vi "dlgTVEFeRFePlot.vi"(8 "error in (no error)":errorcluster, 11 "ResultArray":T1 {"Time Stamp" format="%^<%.3X\n%x>T"}) -> (0 "error out":errorcluster)   [LabVIEW 2014]
uses:
  typedefs/PlotSource.ctl
  typedefs/ResultArray.ctl
  typedefs/Result.ctl
  typedefs/TVE_Fe_RFE.ctl
  typedefs/eMainAction.ctl
panel:
  out "TVE Fe RFe Plot":T4(graph)
  in  "btnExit":bool
  in  "PlotSource":T5
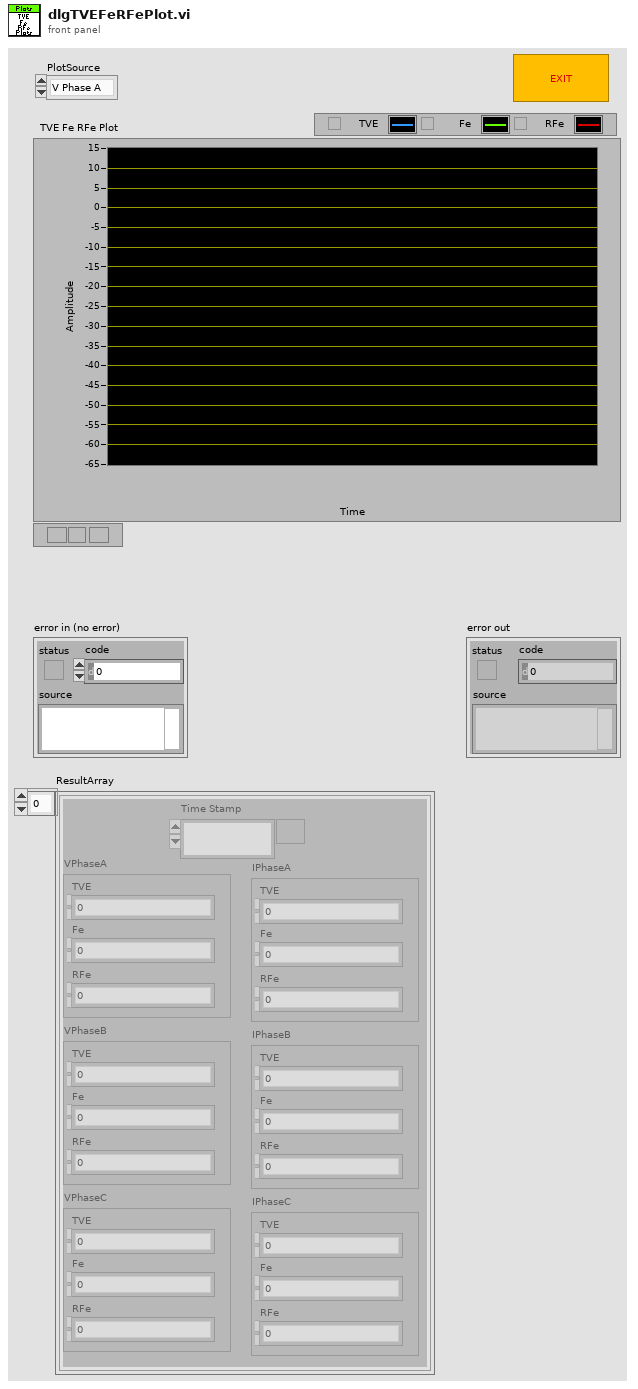
[diagram p1: front panel]
types:
  T1 = typedef "ResultArray.ctl" = T2[]
  T2 = typedef "Result.ctl" = cluster{"Time Stamp":timestamp, "VPhaseA":T3, "VPhaseB":T3, "VPhaseC":T3, "IPhaseA":T3, "IPhaseB":T3, "IPhaseC":T3}
  T3 = typedef "TVE_Fe_RFE.ctl" = cluster{"TVE":dbl, "Fe":dbl, "RFe":dbl}
  T4 = cluster{"TimestampArray":timestamp[], "Y":dbl[]}[]
  T5 = typedef "PlotSource.ctl" = enum16{"V Phase A", "V Phase B", "V Phase C", "I Phase A", "I Phase B", "I Phase C"}
  T6 = typedef "eMainAction.ctl" = enum16{"Init", "ProcessUI", "Exit"}
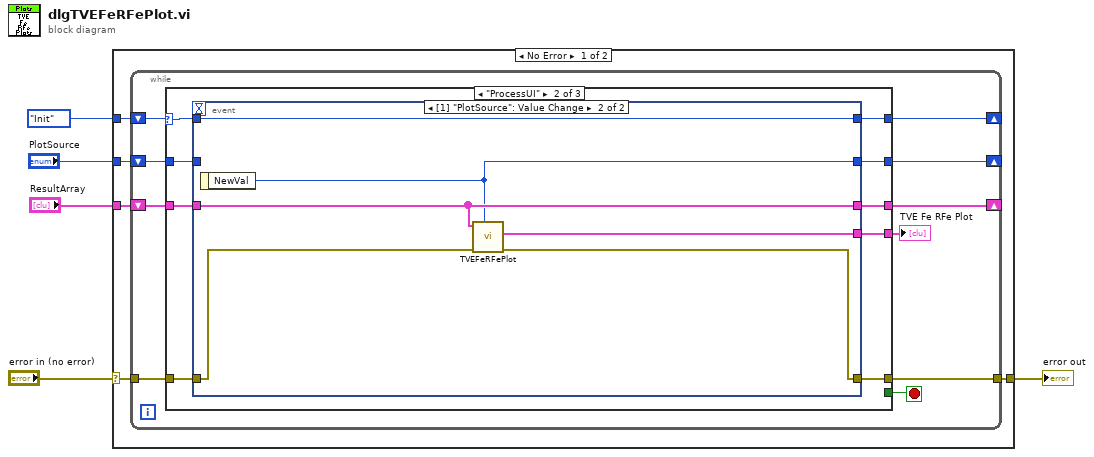
[diagram p0: block diagram]
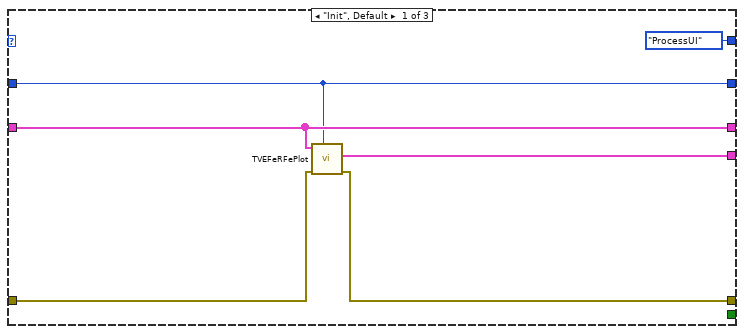
[diagram p2: hidden frame]
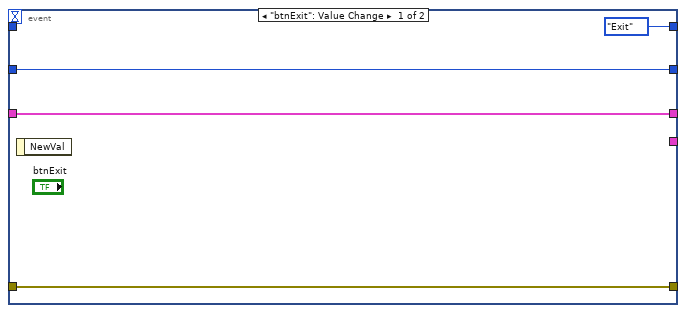
[diagram p3: hidden frame]
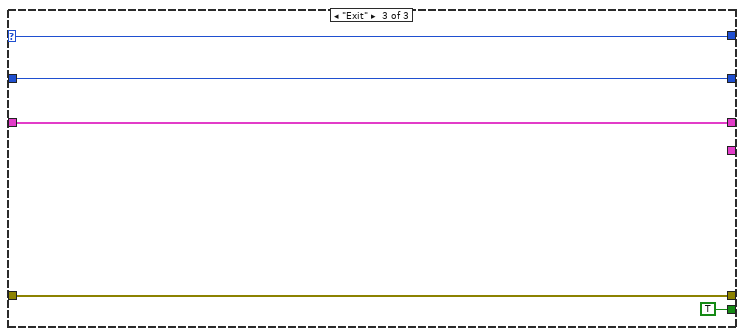
[diagram p4: hidden frame]
diagram:
  n1 = case shown="No Error" "error in (no error)" {
    selector: "error in (no error)" -> [w7 w51]
    tunnel: [w6 w51] -> w4
    tunnel: eMainAction."Init" ("eMainAction") -> [w10 _]
    tunnel: "PlotSource" -> [w9 _]
    tunnel: "ResultArray" -> [w8 _]
    frame No Error {
      n2 = while {
        shift-right: [w19] -> _
        shift-left: w10 -> [w20]
        shift-right: [w15] -> _
        shift-left: w9 -> [w18]
        shift-right: [w16] -> _
        shift-left: w8 -> [w17]
        tunnel: w7 -> [w14]
        tunnel: [w13] -> w6
        stop <- w12 stop-if-true
        n3 = case shown="\"ProcessUI\"" w20 {
          selector: w20 -> [_ w34 w50]
          tunnel: [eMainAction."ProcessUI" ("eMainAction") w35 w50] -> w19
          tunnel: w18 -> [w21 w30 w49]
          tunnel: w17 -> [w23 w32 w48]
          tunnel: [w23 w33 w48] -> w16
          tunnel: [w21 w31 w49] -> w15
          tunnel: w14 -> [w25 w29 w47]
          tunnel: [w24 w28 w47] -> w13
          tunnel: [_ _ TRUE] -> w12
          tunnel: [w22 w27 _] -> w11
          frame "Init", Default {
            n4 = call "TVEFeRFePlot.vi"("PlotSource"=w21, "error in (no error)"=w25, "ResultArray"=w23) -> ("error out"=w24:errorcluster, "TVE Fe RFe Plot"=w22:T4)  [unwired: 7 in]
          }
          frame "ProcessUI" {
            n5 = event shown="[1] \"PlotSource\": Value Change" {
              selector: _ -> [_ _]
              dyn-events: _ -> [_ _]
              timeout: _ -> [_ _]
              tunnel: [eMainAction."Exit" ("eMainAction") w40] -> w35
              tunnel: w34 -> [_ w40]
              tunnel: [w39 w45] -> w33
              tunnel: w32 -> [w39 w45]
              tunnel: [w37 w41] -> w31
              tunnel: w30 -> [w37 _]
              tunnel: w29 -> [w36 w44]
              tunnel: [w36 w42] -> w28
              tunnel: [_ w43] -> w27
              event "btnExit": Value Change {
                n6 = event-data() -> ()  [unwired: 1 in, 1 out]
              }
              event Value Change {
                n7 = event-data() -> ("NewVal"=w41:T5)  [unwired: 1 in]
                n8 = call "TVEFeRFePlot.vi"("PlotSource"=w41, "error in (no error)"=w44, "ResultArray"=w45) -> ("error out"=w42:errorcluster, "TVE Fe RFe Plot"=w43:T4)  [unwired: 7 in]
              }
            }
          }
          frame "Exit" {
          }
        }
        "TVE Fe RFe Plot" <- w11
      }
    }
    frame Error {
    }
  }
  "error out" <- w4
